vi "Fibonacci.vi"() -> ()   [LabVIEW 2024]
panel:
  out "Numero de iteración":i32
  out "Arreglo de salida":i32[](array[numeric])
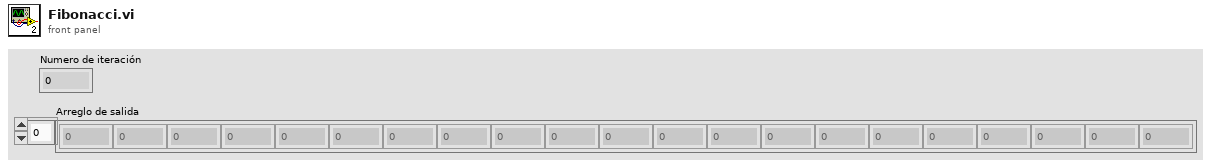
[diagram p1: front panel]
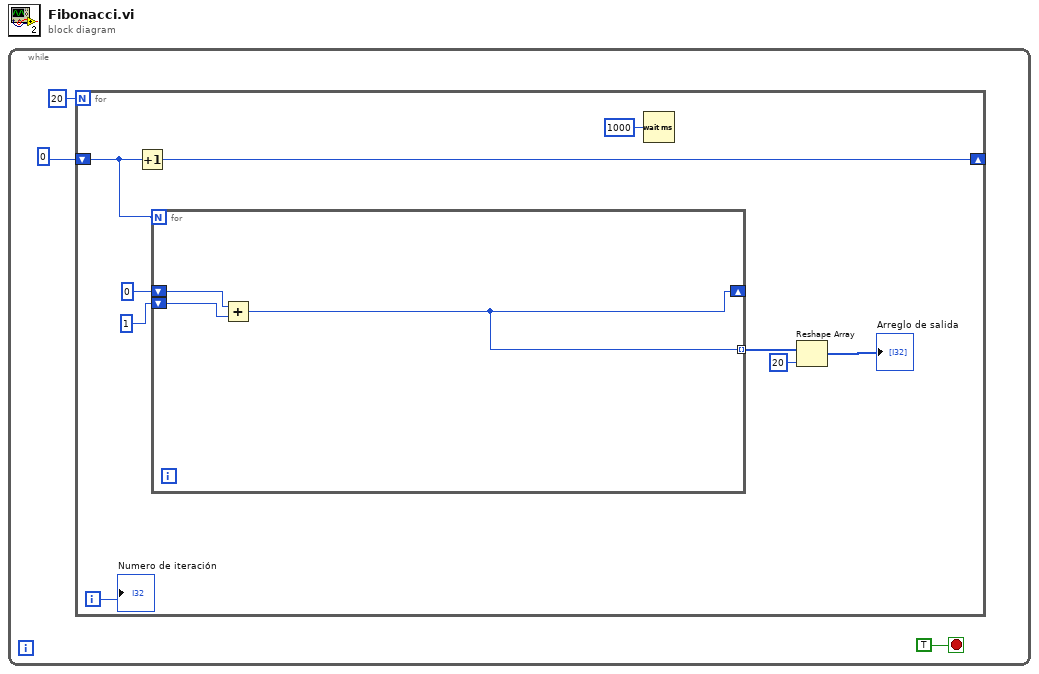
[diagram p0: block diagram]
diagram:
  n1 = while {
    stop <- TRUE stop-if-true
    n2 = for {
      N: 20 -> [_]
      shift-right: [w6] -> _
      shift-left: 0 -> [w5]
      i -> [w4]
      n3 = Increment(x=w5) -> (x+1=w6:i32)
      n4 = for {
        N: w5 -> [_]
        shift-right: [w13] -> _
        shift-left: 0 -> [w15]
        shift-left: 1 -> [w14]
        tunnel: [w13] -> w9 mode=indexing
        n5 = Add(x=w15, y=w14) -> (x+y=w13:i32)
      }
      n6 = Wait (ms)(milliseconds to wait=u32 1000) -> ()  [unwired: 1 out]
      n7 = Reshape Array(w9, 20 ("dimension size")) -> (→"Arreglo de salida":i32[])
      "Numero de iteración" <- w4
    }
  }
